vi "Revision Query.vi"(8 "error in (no error)":errorcluster, 11 "VISA resource name":refnum<visa-resource-name>) -> (0 "error out":errorcluster, 1 "Instrument Firmware Revision":string, 2 "Instrument Driver Revision":string, 3 "VISA resource name out":refnum<visa-resource-name>)   [LabVIEW 2015, in "Voltech PM1000+.lvlib"]
doc: "Queries the current instrument firmware revision and instrument driver revision.\n\nRefer to the Readme file for detailed driver information including modification history."
uses:
  <instrlib>/Voltech PM1000+/Voltech PM1000+.lvlib
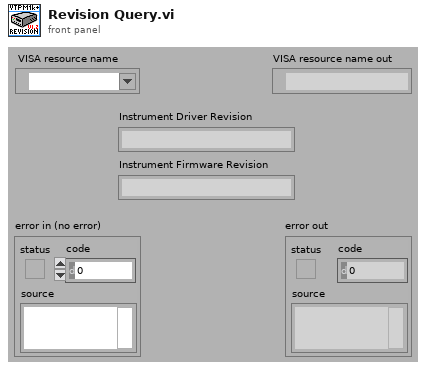
[diagram p1: front panel]
types:
  T1 = enum32{"invalid app kind", "Development System", "Run Time System", "Student Edition", "Embedded LabVIEW", "Evaluation", "Custom"}
  T2 = cluster{"Major":u16, "Minor":u16, "Fix":u16, "Build":u16}
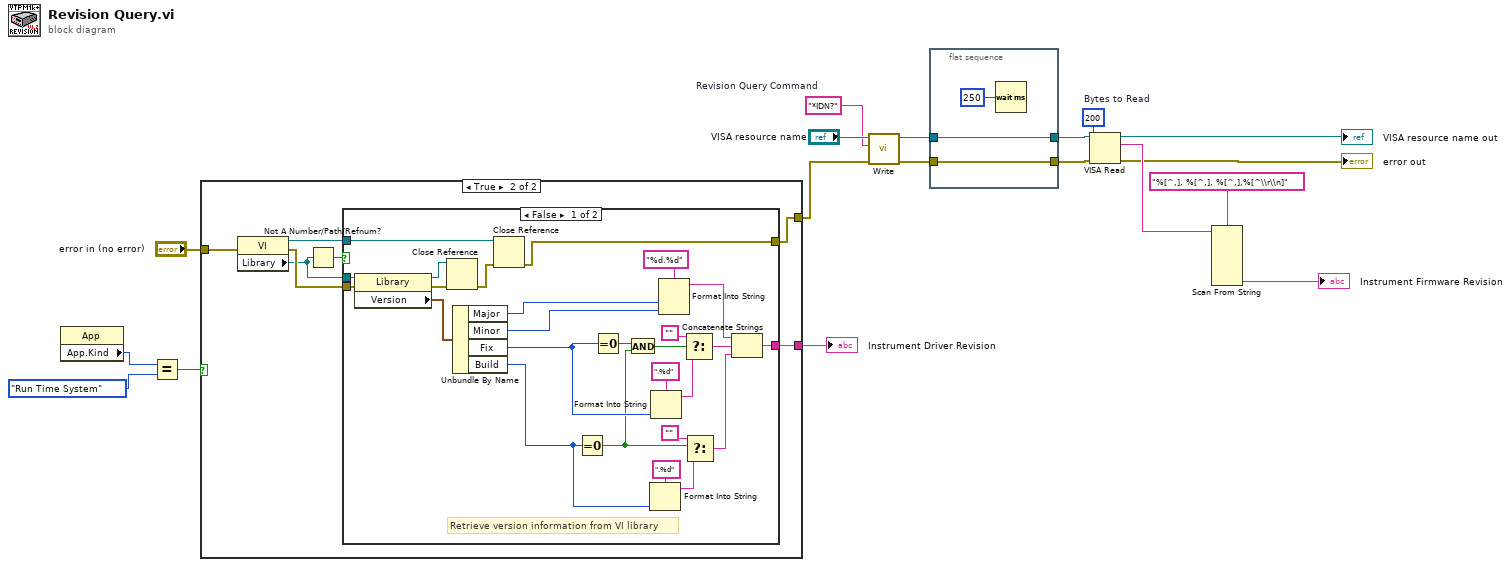
[diagram p0: block diagram]
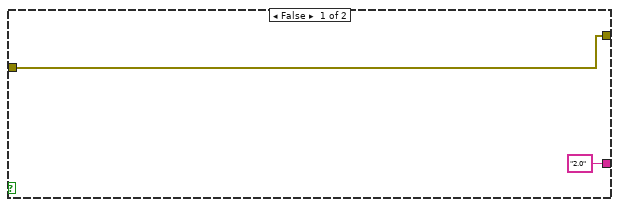
[diagram p2: hidden frame]
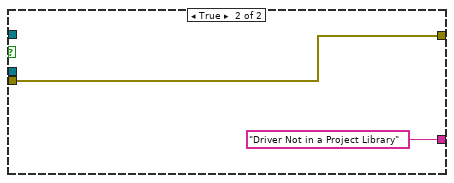
[diagram p3: hidden frame]
diagram:
  w5 = "*IDN?"  # Revision Query Command
  w16 = u32 200  # Bytes to Read
  n1 = property class="App"() -> ("App.Kind"=w3:T1)  [unwired: 2 in, 2 out]
  n2 = Equal?(x=w3, y=T1."Run Time System" ("Application:Kind")) -> (x = y?=w1:bool)
  n3 = case shown="True" w1 {
    tunnel: ["2.0" w23] -> w13
    tunnel: "error in (no error)" -> [w19 w22]
    tunnel: [w19 w21] -> w12
    frame False {
    }
    frame True {
      n4 = property class="VI"(error in=w22) -> (reference out=w27:refnum<vi>, error out=w26:errorcluster, "Library"=w25:refnum<vi>)  [unwired: 1 in]
      n5 = Not A Number/Path/Refnum?(number/path/refnum=w25) -> (NaN/Path/Refnum?=w24:bool)
      n6 = case shown="False" w24 {
        tunnel: w27 -> [w50 _]
        tunnel: w26 -> [w35 w55]
        tunnel: [w30 w55] -> w21
        tunnel: [w29 "Driver Not in a Project Library"] -> w23
        tunnel: w25 -> [w28 _]
        frame False {
          # "Retrieve version information from VI library"
          n7 = property class="Library"(reference=w28, error in=w35) -> (reference out=w52:refnum<vi>, error out=w53:errorcluster, "Version"=w49:T2)
          n8 = Close Reference(reference=w52, error in (no error)=w53) -> (error out=w51:errorcluster)
          n9 = Unbundle By Name(w49) -> ("Major"=w38:u16, "Minor"=w37:u16, "Fix"=w34:u16, "Build"=w36:u16)
          n10 = Close Reference(reference=w50, error in (no error)=w51) -> (error out=w30:errorcluster)
          n11 = Equal To 0?(x=w36) -> (x = 0?=w32:bool)
          n12 = Equal To 0?(x=w34) -> (x = 0?=w33:bool)
          n13 = And(x=w33, y=w32) -> (x .and. y?=w31:bool)
          n14 = Format Into String(format string=".%d", w36) -> (resulting string=w42:string)  [unwired: 2 in, 1 out]
          n15 = Format Into String(format string=".%d", w34) -> (resulting string=w46:string)  [unwired: 2 in, 1 out]
          n16 = Format Into String(format string="%d.%d", w38, w37) -> (resulting string=w44:string)  [unwired: 2 in, 1 out]
          n17 = Select(t="", s=w31, f=w46) -> (s? t:f=w43:string)
          n18 = Select(t="", s=w32, f=w42) -> (s? t:f=w39:string)
          n19 = Concatenate Strings(w44, w43, w39) -> (w29:string)
        }
        frame True {
        }
      }
    }
  }
  "Instrument Driver Revision" <- w13
  n20 = call <instrlib>:"Write.vi"("error in (no error)"=w12, "Write Buffer"=w5, "VISA resource name"="VISA resource name") -> ("error out"=w9:errorcluster, "VISA resource name out"=w7:refnum<visa-resource-name>)  [unwired: 7 in]
  n21 = flat-sequence {
    tunnel: [w58] -> w8
    tunnel: w9 -> [w58]
    tunnel: [w57] -> w6
    tunnel: w7 -> [w57]
    frame #0 {
      n22 = Wait (ms)(milliseconds to wait=250) -> ()  [unwired: 1 out]
    }
  }
  n23 = VISA Read(VISA resource name=w6, byte count=w16, error in (no error)=w8) -> (VISA resource name out=→"VISA resource name out":refnum<visa-resource-name>, read buffer=w15:string, error out=→"error out":errorcluster)  [unwired: 1 out]
  n24 = Scan From String(format string="%[^,], %[^,], %[^,],%[^\\r\\n]", input string=w15) -> (output 4=→"Instrument Firmware Revision":string)  [unwired: 9 in, 3 out]
